vi "Stamp off.vi"(11 "Serial Port":refnum<visa-resource-name>) -> (2 "Controls out":T1 {"Pump speed" format="%.2f"}, 3 "Serial Port out":refnum<visa-resource-name>)   [LabVIEW 2012]
uses:
  Stamp Controls.ctl
  switches.ctl
panel:
  out "error out":errorcluster
  # "rpm"
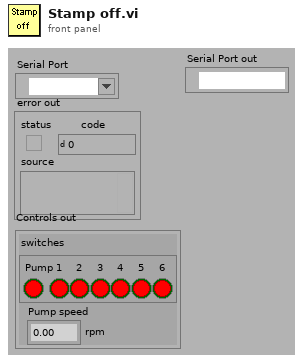
[diagram p1: front panel]
types:
  T1 = typedef "Stamp Controls.ctl" = cluster{"Pump speed":dbl, "switches":T2}
  T2 = typedef "switches.ctl" = cluster{"Pump":bool, "1":bool, "2":bool, "3":bool, "4":bool, "5":bool, "6":bool}
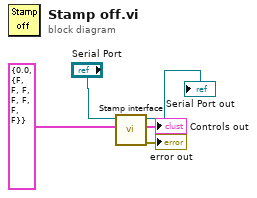
[diagram p0: block diagram]
diagram:
  n1 = call "Stamp interface.vi"("Controls"=T1 {"Pump speed"=0.0, "switches"={"Pump"=FALSE, "1"=FALSE, "2"=FALSE, "3"=FALSE, "4"=FALSE, "5"=FALSE, "6"=FALSE}}, "Serial Port"="Serial Port") -> ("error out"=→"error out":errorcluster, "Controls out"=→"Controls out":T1, "Serial Port out"=→"Serial Port out":refnum<visa-resource-name>)  [unwired: 6 in, 1 out]
